vi "Th_stopwatch_Lap.vi"   [LabVIEW 2018]
uses:
  Th_GUI.vi
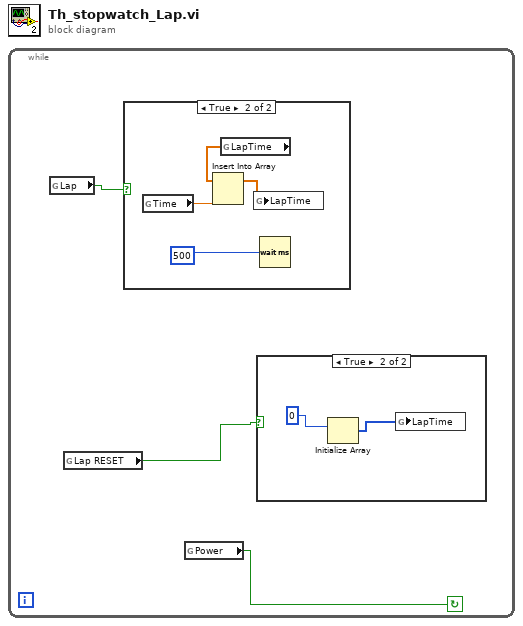
[diagram p0: block diagram]
diagram:
  n1 = while {
    stop <- w1 continue-if-true
    n2 = global read "Th_GUI.vi" "Lap"() -> (w3:bool)
    n3 = global read "Th_GUI.vi" "Lap RESET"() -> (w2:bool)
    n4 = case shown="TRUE" w3 {
      frame False {
      }
      frame True {
        n5 = global read "Th_GUI.vi" "Time"() -> (w7:dbl)
        n6 = global read "Th_GUI.vi" "LapTime"() -> (w9:dbl[])
        n7 = Insert Into Array(array=w9, new element=w7) -> (w8:dbl[])  [unwired: 1 in]
        n8 = global write "Th_GUI.vi" "LapTime"(w8) -> ()
        n9 = Wait (ms)(milliseconds to wait=500) -> ()  [unwired: 1 out]
      }
    }
    n10 = global read "Th_GUI.vi" "Power"() -> (w1:bool)
    n11 = case shown="TRUE" w2 {
      frame False {
      }
      frame True {
        n12 = Initialize Array(0) -> (w4:i32[])  [unwired: 1 in]
        n13 = global write "Th_GUI.vi" "LapTime"(w4) -> ()
      }
    }
  }
